vi "InsertHorizontalLine.vi"(8 "error in (no error)":errorcluster, 10 "ParentTag":string, 11 "MGI_TrayIcon in":refnum<class "MGI_TrayIcon.lvclass">) -> (0 "error out":errorcluster, 3 "MGI_TrayIcon out":refnum<class "MGI_TrayIcon.lvclass">)   [LabVIEW 2016, in "MGI_TrayIcon.lvclass"]
doc: "Authored by Derek E. Trepanier\nsupport@mooregoodideas.com\nwww.mooregoodideas.com\n\nCopyright (c) 2012, Moore Good Ideas, Inc.\n\nAll rights reserved.\n\nRedistribution and use in source and binary forms, with or without modification, are permitted provided that the following conditions are met:\n\n * Redistributions of source code must retain the above copyright notice, this list of conditions and the following disclaimer.\n * Redistributions in binary form must reproduce the above copyright notice, this list of conditions and the following disclaimer in the documentation and/or other materials provided with the distribution.\n * Neither the name of Moore Good Ideas, Inc. nor the names of its contributors may be used to endorse or promote products derived from this software without specific prior written permission.\n\nTHIS SOFTWARE IS PROVIDED BY THE COPYRIGHT HOLDERS AND CONTRIBUTORS \"AS IS\" AND ANY EXPRESS OR IMPLIED WARRANTIES, INCLUDING, BUT NOT LIMITED TO, THE IMPLIED WARRANTIES OF MERCHANTABILITY AND FITNESS FOR A PARTICULAR PURPOSE ARE DISCLAIMED. IN NO EVENT SHALL THE COPYRIGHT OWNER OR CONTRIBUTORS BE LIABLE FOR ANY DIRECT, INDIRECT, INCIDENTAL, SPECIAL, EXEMPLARY, OR CONSEQUENTIAL DAMAGES (INCLUDING, BUT NOT LIMITED TO, PROCUREMENT OF SUBSTITUTE GOODS OR SERVICES; LOSS OF USE, DATA, OR PROFITS; OR BUSINESS INTERRUPTION) HOWEVER CAUSED AND ON ANY THEORY OF LIABILITY, WHETHER IN CONTRACT, STRICT LIABILITY, OR TORT (INCLUDING NEGLIGENCE OR OTHERWISE) ARISING IN ANY WAY OUT OF THE USE OF THIS SOFTWARE, EVEN IF ADVISED OF THE POSSIBILITY OF SUCH DAMAGE."
uses:
  <userlib>/_MGI/Menu Building/MenuTypes/TrayIcon/MGI_TrayIcon.lvclass
  <userlib>/_MGI/Menu Building/MenuTypes/TrayIcon/MGI_TrayIcon.lvclass/MGI_TrayIcon.ctl
  System.Windows.Forms
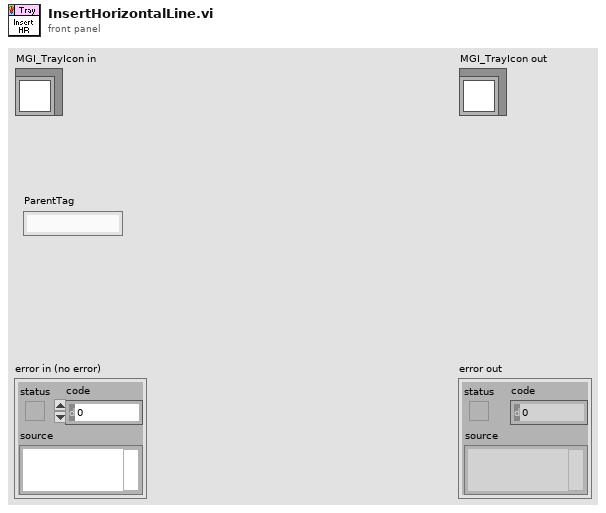
[diagram p1: front panel]
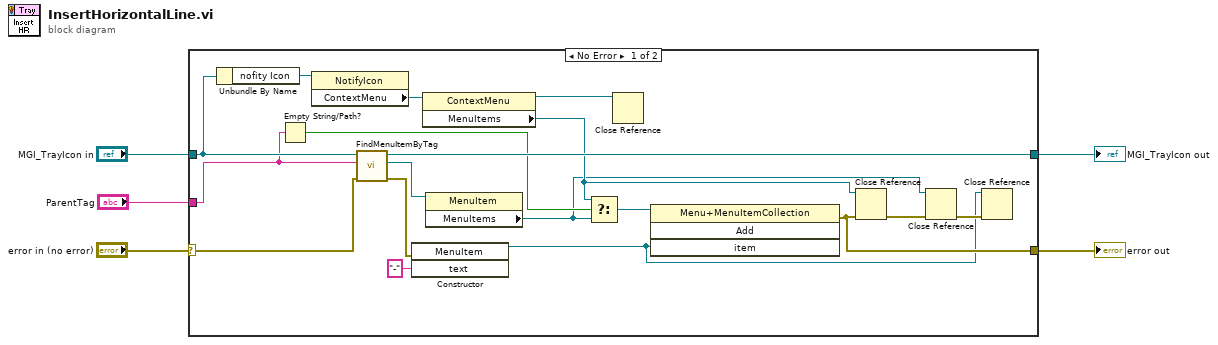
[diagram p0: block diagram]
diagram:
  n1 = case shown="No Error" "error in (no error)" {
    selector: "error in (no error)" -> [w22 w24]
    tunnel: "MGI_TrayIcon in" -> [w16 w25]
    tunnel: [w23 w25] -> w4
    tunnel: "ParentTag" -> [w14 _]
    tunnel: [w11 w24] -> w1
    frame No Error {
      n2 = Unbundle By Name(w16) -> ("nofity Icon"=w18:refnum<k24>)
      n3 = Empty String/Path?(string/path=w14) -> (empty?=w13:bool)
      n4 = property class="NotifyIcon"(reference=w18) -> ("ContextMenu"=w17:refnum<k24>)  [unwired: 1 in, 2 out]
      n5 = call <userlib>:"FindMenuItemByTag.vi"("error in (no error)"=w22, "Full Tag"=w14, "NotifyIcon in"=w16) -> ("error out"=w19:errorcluster, "Menu Item"=w21:refnum<k24>, "NotifyIcon out"=w23:refnum<class "MGI_TrayIcon.lvclass">)  [unwired: 6 in]
      n6 = constructor class="MenuItem"(error in=w19, "text"="-") -> (reference out=w6:refnum<k24>)  [unwired: 2 in, 3 out]
      n7 = property class="ContextMenu"(reference=w17) -> (reference out=w12:refnum<k24>, "MenuItems"=w10:refnum<k24>)  [unwired: 1 in, 1 out]
      n8 = property class="MenuItem"(reference=w21) -> ("MenuItems"=w8:refnum<k24>)  [unwired: 1 in, 2 out]
      n9 = Select(t=w10, s=w13, f=w8) -> (s? t:f=w15:refnum<k24>)
      n10 = Close Reference(reference=w12) -> ()  [unwired: 1 in, 1 out]
      n11 = invoke class="Menu+MenuItemCollection" method="Add"(reference=w15, "item"=w6) -> (error out=w11:errorcluster)  [unwired: 2 in, 3 out]
      n12 = Close Reference(reference=w10, error in (no error)=w11) -> (error out=w9:errorcluster)
      n13 = Close Reference(reference=w8, error in (no error)=w9) -> (error out=w7:errorcluster)
      n14 = Close Reference(reference=w6, error in (no error)=w7) -> ()  [unwired: 1 out]
    }
    frame Error {
    }
  }
  "error out" <- w1
  "MGI_TrayIcon out" <- w4
